vi "#111_MAV_MSG_TIMESYNC.vi"(11 "mavlink_payload":u8[](array[numeric])) -> (3 "TIMESYNC":T1)   [LabVIEW 2023]
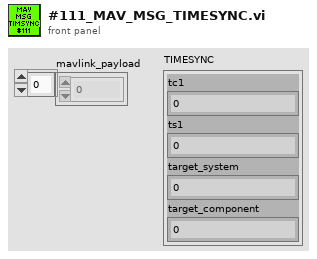
[diagram p1: front panel]
types:
  T1 = cluster{"tc1":i64, "ts1":i64, "target_system":u8, "target_component":u8}
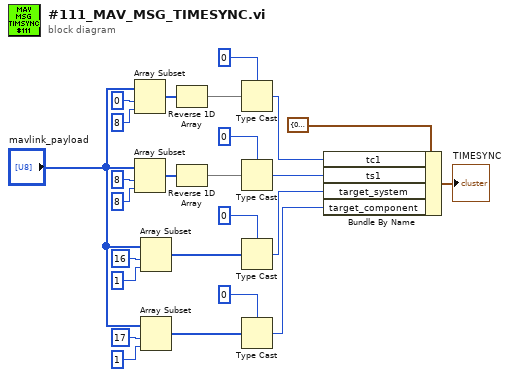
[diagram p0: block diagram]
diagram:
  n1 = Array Subset(array="mavlink_payload", index=0 ("Index"), length=8) -> (w24:u8[])
  n2 = Array Subset(array="mavlink_payload", index=8 ("Index"), length=8) -> (w16:u8[])
  n3 = Array Subset(array="mavlink_payload", index=16 ("Index"), length=1) -> (w8:u8[])
  n4 = Array Subset(array="mavlink_payload", index=17 ("Index"), length=1) -> (w4:u8[])
  n5 = Reverse 1D Array(array=w24) -> (reversed array=w23:u8[])
  n6 = Reverse 1D Array(array=w16) -> (reversed array=w15:u8[])
  n7 = Type Cast(type=i64 0 ("Index"), x=w23) -> (*(type *) &x=w18:i64)
  n8 = Type Cast(type=i64 0 ("Index"), x=w15) -> (*(type *) &x=w12:i64)
  n9 = Type Cast(type=u8 0 ("Index"), x=w8) -> (*(type *) &x=w2:u8)
  n10 = Type Cast(type=u8 0 ("Index"), x=w4) -> (*(type *) &x=w1:u8)
  n11 = Bundle By Name(cluster=T1 {"tc1"=0, "ts1"=0, "target_system"=0, "target_component"=0} ("TIMESYNC"), "tc1"=w18, "ts1"=w12, "target_system"=w2, "target_component"=w1) -> (→"TIMESYNC":T1)
